vi "Read Joystick.vi"(8 "Joystick Deadbanded Value (default of 0.1)":dbl, 10 "Joystick R 2 DevRef":T1, 11 "Joystick L 1 DevRef":T1) -> (0 "Wheel Lock":bool=TRUE, 1 "Joystick R 2 X Axis":dbl, 2 "Joystick L 1 Y Axis":dbl, 3 "Joystick L 1 X Axis":dbl, 4 "Radial Spin":bool, 6 "axis 3 (throttle)":dbl)   [LabVIEW 2012]
uses:
  <vilib>/Rock Robotics/WPI/Joystick/WPI_JoystickDevRef.ctl
  <vilib>/Rock Robotics/WPI/Joystick/WPI_JoystickDeviceEnum.ctl
  Begin/Global Variables.vi
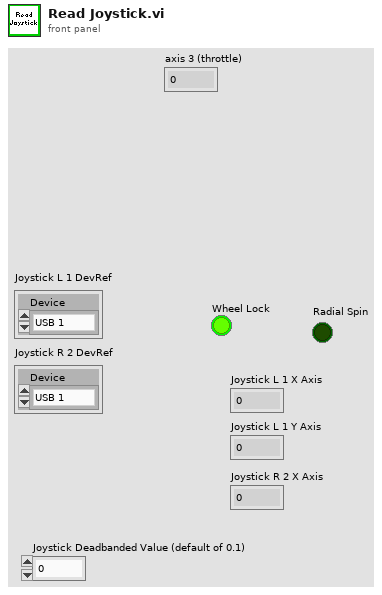
[diagram p1: front panel]
types:
  T1 = typedef "WPI_JoystickDevRef.ctl" = cluster{"Device":T2}
  T2 = typedef "WPI_JoystickDeviceEnum.ctl" = enum16{"USB 1", "USB 2", "USB 3", "USB 4", "Kinect 1", "Kinect 2"}
  T3 = typedef "WPI_JoystickButtonState.ctl" = cluster{"Button 1":bool, "Button 2":bool, "Button 3":bool, "Button 4":bool, "Button 5":bool, "Button 6":bool, "Button 7":bool, "Button 8":bool, "Button 9":bool, "Button 10":bool, "Button 11":bool, "Button 12":bool}
  T4 = cluster{"axis 1 (x)":dbl, "axis 2 (y)":dbl, "axis 3 (throttle)":dbl, "axis 4":dbl, "axis 5":dbl, "axis 6":dbl}
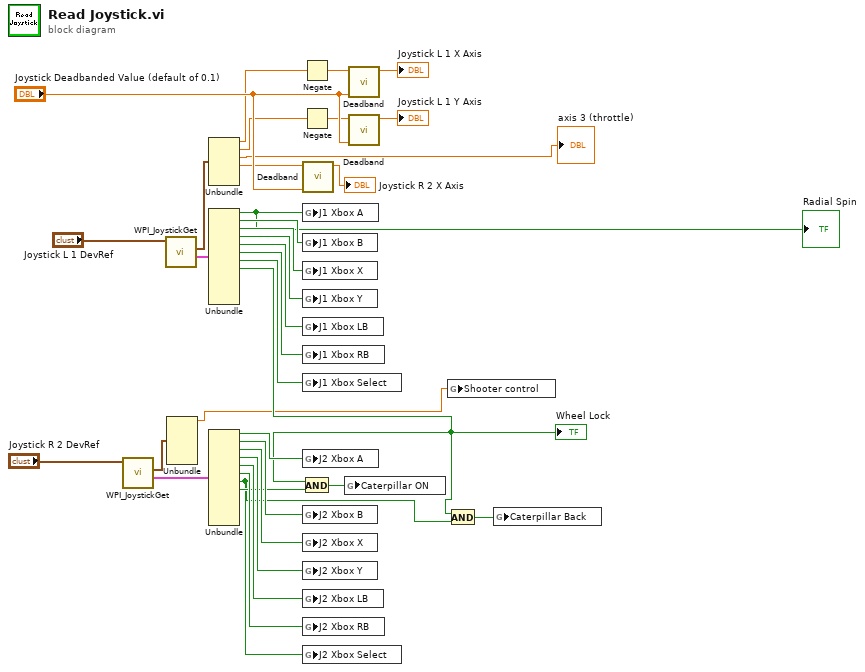
[diagram p0: block diagram]
diagram:
  n1 = call <vilib>:"WPI_JoystickGet.vi"("JoystickDevRef"="Joystick R 2 DevRef") -> ("Buttons"=w25:T3, "Axes"=w24:T4)  [unwired: 4 in, 1 out]
  n2 = call <vilib>:"WPI_JoystickGet.vi"("JoystickDevRef"="Joystick L 1 DevRef") -> ("Buttons"=w35:T3, "Axes"=w34:T4)  [unwired: 4 in, 1 out]
  n3 = Unbundle(w24) -> ("axis 1 (x)"=w2:dbl)  [unwired: 5 out]
  n4 = Unbundle(w34) -> ("axis 1 (x)"=w18:dbl, "axis 2 (y)"=w28:dbl, "axis 3 (throttle)"=→"axis 3 (throttle)":dbl, "axis 4"=w10:dbl)  [unwired: 2 out]
  n5 = Unbundle(w35) -> ("Button 1"=w3:bool, "Button 2"=w14:bool, "Button 3"=w20:bool, "Button 4"=w16:bool, "Button 5"=w26:bool, "Button 6"=w27:bool, "Button 7"=w8:bool, "Button 8"=w5:bool)  [unwired: 4 out]
  "Wheel Lock" <- w5
  "Radial Spin" <- w3
  n6 = Unbundle(w25) -> ("Button 1"=w22:bool, "Button 2"=w12:bool, "Button 3"=w15:bool, "Button 4"=w13:bool, "Button 5"=w21:bool, "Button 6"=w11:bool, "Button 7"=w4:bool, "Button 8"=w7:bool)  [unwired: 4 out]
  n7 = Negate(x=w18) -> (-x=w19:dbl)
  n8 = Negate(x=w28) -> (-x=w17:dbl)
  n9 = And(x=w5, y=w7) -> (x .and. y?=w9:bool)
  n10 = call "Deadband.vi"("Value to Deadband (default of 0.1)"="Joystick Deadbanded Value (default of 0.1)", "Value"=w10) -> ("Deadbanded Value"=→"Joystick R 2 X Axis":dbl)  [unwired: 9 in]
  n11 = global write "Global Variables.vi" "J1 Xbox A"(w3) -> ()
  n12 = global write "Global Variables.vi" "J1 Xbox B"(w14) -> ()
  n13 = global write "Global Variables.vi" "J1 Xbox X"(w20) -> ()
  n14 = global write "Global Variables.vi" "J1 Xbox Y"(w16) -> ()
  n15 = global write "Global Variables.vi" "J1 Xbox LB"(w26) -> ()
  n16 = global write "Global Variables.vi" "J1 Xbox RB"(w27) -> ()
  n17 = global write "Global Variables.vi" "J1 Xbox Select"(w8) -> ()
  n18 = global write "Global Variables.vi" "J2 Xbox A"(w22) -> ()
  n19 = global write "Global Variables.vi" "J2 Xbox B"(w12) -> ()
  n20 = global write "Global Variables.vi" "J2 Xbox X"(w15) -> ()
  n21 = global write "Global Variables.vi" "J2 Xbox Y"(w13) -> ()
  n22 = global write "Global Variables.vi" "J2 Xbox LB"(w21) -> ()
  n23 = global write "Global Variables.vi" "J2 Xbox RB"(w11) -> ()
  n24 = global write "Global Variables.vi" "J2 Xbox Select"(w4) -> ()
  n25 = global write "Global Variables.vi" "Caterpillar ON"(w9) -> ()
  n26 = call "Deadband.vi"("Value to Deadband (default of 0.1)"="Joystick Deadbanded Value (default of 0.1)", "Value"=w19) -> ("Deadbanded Value"=→"Joystick L 1 X Axis":dbl)  [unwired: 9 in]
  n27 = call "Deadband.vi"("Value to Deadband (default of 0.1)"="Joystick Deadbanded Value (default of 0.1)", "Value"=w17) -> ("Deadbanded Value"=→"Joystick L 1 Y Axis":dbl)  [unwired: 9 in]
  n28 = global write "Global Variables.vi" "Shooter control"(w2) -> ()
  n29 = And(x=w5, y=w4) -> (x .and. y?=w6:bool)
  n30 = global write "Global Variables.vi" "Caterpillar Back"(w6) -> ()
